vi "Close.vi"(8 "error in (no error)":errorcluster, 11 "NKT in":refnum<class "NKT_Extreme.lvclass">) -> (0 "error out":errorcluster, 3 "NKT out":refnum<class "NKT_Extreme.lvclass">)   [LabVIEW 2020, in "NKT_Extreme.lvclass"]
uses:
  <instrlib>/Classes/Laser/NKT/NKT_Extreme.lvclass
  <instrlib>/NKTP_API/NKTP_API.lvlib
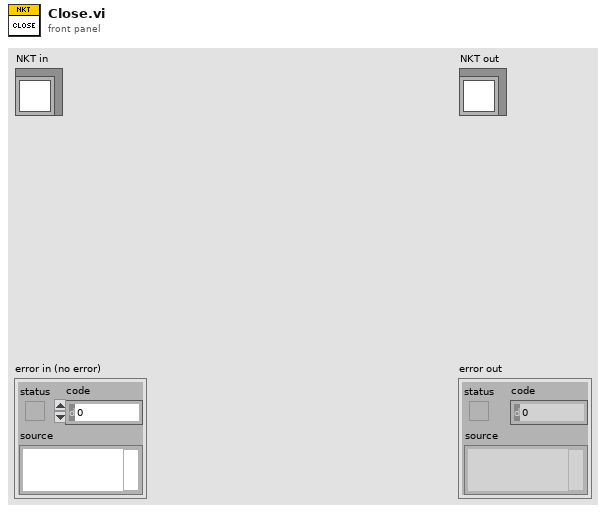
[diagram p1: front panel]
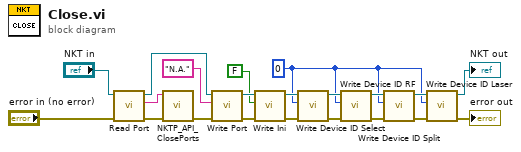
[diagram p0: block diagram]
diagram:
  w3 = u8 0 ("Device ID Select")
  n1 = call-dynamic "Read Port.vi"("error in (no error)"="error in (no error)", "NKT in"="NKT in") -> ("error out"=w18:errorcluster, "Port"=w19:string, "NKT out"=w17:refnum<class "NKT_Extreme.lvclass">)  [unwired: 7 in]
  n2 = call <instrlib>:"NKTP_API_ClosePorts.vi"("error in"=w18, "portnames"=w19) -> ("error out"=w16:errorcluster)  [unwired: 8 in, 1 out]
  n3 = call-dynamic "Write Port.vi"("error in (no error)"=w16, "Port"="N.A.", "NKT in"=w17) -> ("error out"=w15:errorcluster, "NKT out"=w14:refnum<class "NKT_Extreme.lvclass">)  [unwired: 7 in]
  n4 = call-dynamic "Write Ini.vi"("error in (no error)"=w15, "Init"=FALSE, "NKT in"=w14) -> ("error out"=w11:errorcluster, "NKT out"=w10:refnum<class "NKT_Extreme.lvclass">)  [unwired: 7 in]
  n5 = call-dynamic "Write Device ID Select.vi"("error in (no error)"=w11, "Device ID Select"=w3, "NKT in"=w10) -> ("error out"=w9:errorcluster, "NKT out"=w8:refnum<class "NKT_Extreme.lvclass">)  [unwired: 7 in]
  n6 = call-dynamic "Write Device ID RF.vi"("error in (no error)"=w9, "Device ID RF"=w3, "NKT in"=w8) -> ("error out"=w7:errorcluster, "NKT out"=w6:refnum<class "NKT_Extreme.lvclass">)  [unwired: 7 in]
  n7 = call-dynamic "Write Device ID Split.vi"("error in (no error)"=w7, "Device ID Split"=w3, "NKT in"=w6) -> ("error out"=w5:errorcluster, "NKT out"=w4:refnum<class "NKT_Extreme.lvclass">)  [unwired: 7 in]
  n8 = call-dynamic "Write Device ID Laser.vi"("error in (no error)"=w5, "Device ID Laser"=w3, "NKT in"=w4) -> ("error out"=→"error out":errorcluster, "NKT out"=→"NKT out":refnum<class "NKT_Extreme.lvclass">)  [unwired: 7 in]
